vi "strip final segment of an IP address.vi"(11 "1st column 1st data":string[](array[string])) -> (3 "Output Array":string[](array[string]))   [LabVIEW 2020]
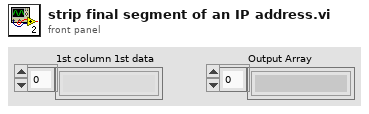
[diagram p1: front panel]
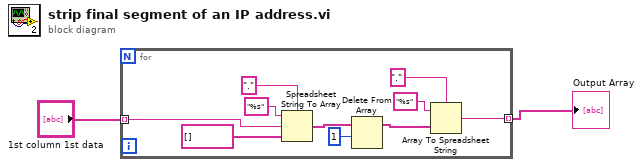
[diagram p0: block diagram]
diagram:
  n1 = for {
    tunnel: "1st column 1st data" -> [w11] mode=indexing
    tunnel: [w5] -> w1 mode=indexing
    n2 = Spreadsheet String To Array(delimiter (Tab)=".", format string="%s", spreadsheet string=w11, array type (2D Dbl)=string[] [] ("1st column 1st data")) -> (array=w9:string[])
    n3 = Delete From Array(array=w9, length=1) -> (array with subset deleted=w7:string[])  [unwired: 1 in, 1 out]
    n4 = Array To Spreadsheet String(delimiter (Tab)=".", array=w7, 3:"%s" ("format string")) -> (spreadsheet string=w5:string)
  }
  "Output Array" <- w1
